vi "getTimestamp[]Value.vi"(7 "Name":string, 8 "error in (no error)":errorcluster, 11 "tBSONDocument in":refnum<class "tBSONDocument.lvclass">) -> (0 "error out":errorcluster, 2 "Value":timestamp[](array[timestamp]), 3 "tBSONDocument out":refnum<class "tBSONDocument.lvclass">)   [LabVIEW 2013, in "BSON.lvlib" / "tBSONDocument.lvclass"]
doc: "Retrieves an array of timestamps from a BSON document."
uses:
  tBSONDocument.lvclass
  BSONElements/tBSONArray/tBSONArray.lvclass
  BSONElements/tBSONTimestamp/tBSONTimestamp.lvclass
  BSONElements/tBSONArray/getValue.vi
  BSONElements/tBSONTimestamp/getValue.vi
  tBSONElement/tBSONElement.lvclass
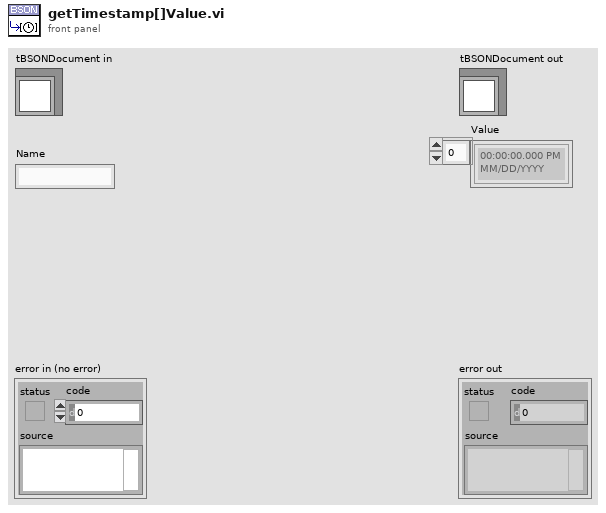
[diagram p1: front panel]
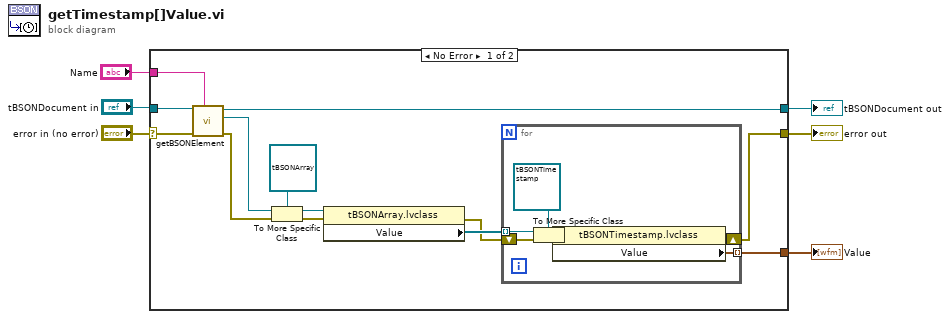
[diagram p0: block diagram]
diagram:
  n1 = case shown="No Error" "error in (no error)" {
    selector: "error in (no error)" -> [w18 w28]
    tunnel: [w9 w28] -> w4
    tunnel: [w17 w27] -> w2
    tunnel: "tBSONDocument in" -> [w19 w27]
    tunnel: "Name" -> [w7 _]
    tunnel: [w8 _] -> w1
    frame No Error {
      n2 = call "getBSONElement.vi"("Name"=w7, "error in (no error)"=w18, "tBSONDocument in"=w19) -> ("error out"=w14:errorcluster, "Element"=w15:refnum<class "tBSONElement.lvclass">, "tBSONDocument out"=w17:refnum<class "tBSONDocument.lvclass">)  [unwired: 6 in]
      n3 = To More Specific Class(target class=refnum<class "tBSONArray.lvclass"> refnum ("BSON.lvlib:tBSONArray.lvclass"), reference=w15, error in=w14) -> (specific class reference=w13:refnum<class "tBSONArray.lvclass">, error out=w12:errorcluster)
      n4 = property class="tBSONArray.lvclass"(reference=w13, error in=w12) -> (error out=w10:errorcluster, "Value"=w11:refnum<class "tBSONElement.lvclass">[])  [unwired: 1 out]
      n5 = for {
        tunnel: w11 -> [w25] mode=indexing
        shift-right: [w22] -> w9
        shift-left: w10 -> [w26]
        tunnel: [w21] -> w8 mode=indexing
        n6 = To More Specific Class(target class=refnum<class "tBSONTimestamp.lvclass"> refnum ("lvMongoDriver.lvlib:BSON.lvlib:tBSONTimestamp.lvclass"), reference=w25, error in=w26) -> (specific class reference=w24:refnum<class "tBSONTimestamp.lvclass">, error out=w23:errorcluster)
        n7 = property class="tBSONTimestamp.lvclass"(reference=w24, error in=w23) -> (error out=w22:errorcluster, "Value"=w21:timestamp)  [unwired: 1 out]
      }
    }
    frame Error {
    }
  }
  "error out" <- w4
  "tBSONDocument out" <- w2
  "Value" <- w1
